vi "Enable and Disable Panel Controls.vi"(3 "VI Reference In":refnum<vi>, 4 "Disabled":T1(ring), 5 "Items to Hide":string[](array[string])) -> (0 "VI Reference Out":refnum<vi>)   [LabVIEW 2016]
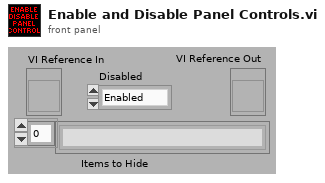
[diagram p1: front panel]
types:
  T1 = enum8{"Enabled", "Disabled", "Disabled and Grayed Out"}
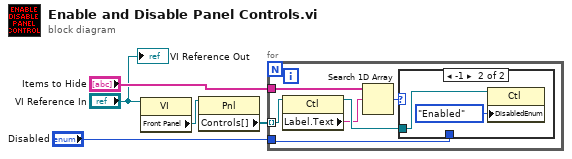
[diagram p0: block diagram]
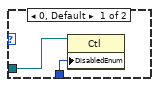
[diagram p2: hidden frame]
diagram:
  n1 = property class="VI"(reference="VI Reference In") -> ("Front Panel"=w4:refnum<vi>)  [unwired: 1 in, 2 out]
  n2 = property class="Pnl"(reference=w4) -> ("Controls[]"=w3:refnum<vi>[])  [unwired: 1 in, 2 out]
  n3 = for {
    tunnel: "Items to Hide" -> [w9]
    tunnel: w3 -> [w11] mode=indexing
    tunnel: "Disabled" -> [w6]
    n4 = property class="Ctl"(reference=w11) -> (reference out=w10:refnum<vi>, "Label.Text"=w8:string)  [unwired: 1 in, 1 out]
    n5 = Search 1D Array(1D array=w9, element=w8) -> (index of element=w7:i32)  [unwired: 1 in]
    n6 = case shown="-1" w7 {
      tunnel: w10 -> [w13 w14]
      tunnel: w6 -> [w12 _]
      frame 0, Default {
        n7 = property class="Ctl"(reference=w13, "DisabledEnum"=w12) -> ()  [unwired: 1 in, 2 out]
      }
      frame -1 {
        n8 = property class="Ctl"(reference=w14, "DisabledEnum"=T1."Enabled" ("Disabled")) -> ()  [unwired: 1 in, 2 out]
      }
    }
  }
  "VI Reference Out" <- "VI Reference In"
